vi "GenericProcess.vi"(11 "YTESTER测试数据":T1 caption="不要修改！") -> (3 "YTESTER结论":T2)   [LabVIEW 2017]
doc: "VIDescription=对某个变量进行判断的简单测试"
uses:
  YtCommon.lvlibp/yt`Step StepBaseInput.ctl
  YtCommon.lvlibp/yt`Step StepResult.ctl
  YtCommon.lvlibp/yt`Step TestData.ctl
  YtCommon.lvlibp/yt`Step System Queue.ctl
  Step`s VIs/YYLLGeneric/variable_W.ctl
  YtCommon.lvlibp/yt`Data-Ytester Type Data.ctl
  YtCommon.lvlibp
panel:
  in  "YTESTER开放参数":T4={"YTESTER_BaseInput"={"isTest"=FALSE, "isSkip"=FALSE, "StepName"="通用简易解析处理", "OnPass"=enum."Next", "OnFail"=enum."Next", "ReTestNumber"=0.0}, "数据源什么类型？"=enum."String类型", "String数据源"="", "NUM数据源"=0.0, "Bool数据源"=FALSE, "Smart预处理"=[], "解析后到变量(自定义建议#开头)"="#YtGenProcess1"}
  # "通用简易解析处理"
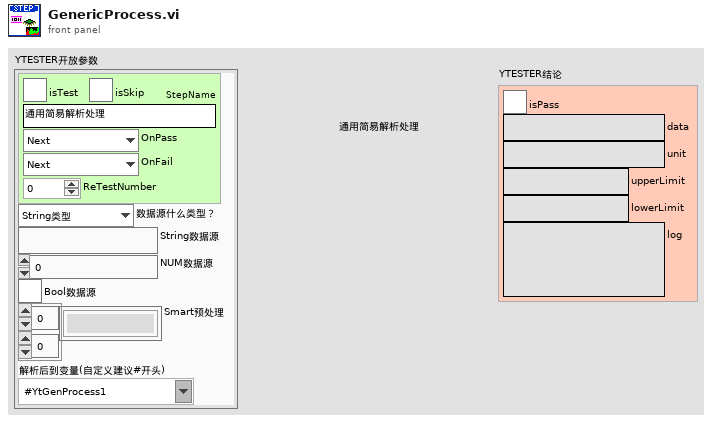
[diagram p1: front panel]
types:
  T1 = typedef "YtCommon.lvlibp/yt`Step TestData.ctl" = cluster{"Socket(From1)":i32, "SN":refnum<notifier>, "StopFlagRef":refnum<notifier>, "YT System Queue":refnum<queue>}
  T2 = typedef "YtCommon.lvlibp/yt`Step StepResult.ctl" = cluster{"isPass":bool, "data":string, "unit":string, "upperLimit":string, "lowerLimit":string, "log":string}
  T3 = typedef "YtCommon.lvlibp/yt`Step StepBaseInput.ctl" = cluster{"isTest":bool, "isSkip":bool, "StepName":string, "OnPass":enum16{"Next", "ToOVER", "Terminate"}, "OnFail":enum16{"Next", "ToOVER", "Terminate"}, "ReTestNumber":dbl}
  T4 = cluster{"YTESTER_BaseInput":T3, "数据源什么类型？":enum16{"String类型", "NUM类型", "Bool类型"}, "String数据源":string, "NUM数据源":dbl, "Bool数据源":bool, "Smart预处理":string[][], "解析后到变量(自定义建议#开头)":string}
  T5 = typedef "variable_W.ctl" = cluster{"YT_TYPE":T6, "TypeData":string[], "Tips":string}
  T6 = typedef "YtCommon.lvlibp/yt`Data-Ytester Type Data.ctl" = enum16{"NULL", "NUM", "BOOL", "TXT", "ENUM", "TIME", "PATH", "VISA", "COMBO", "ColorBox", "RadioBtn", "Array_NUM", "Array_BOOL", "Array_TXT", "Array_ENUM", "Array_PATH", "Array_COMBO"}
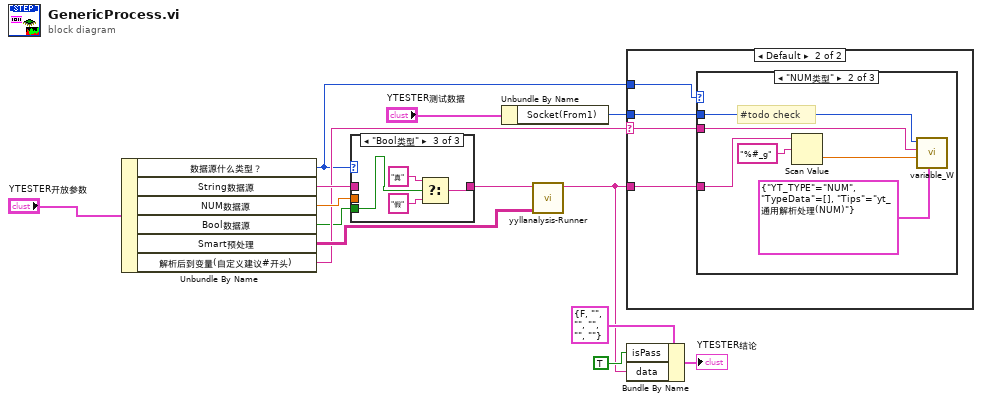
[diagram p0: block diagram]
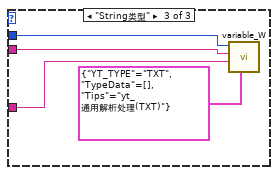
[diagram p4: hidden frame]
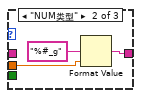
[diagram p6: hidden frame]
diagram:
  # "Y Y L L"
  n1 = Unbundle By Name("YTESTER开放参数") -> ("数据源什么类型？"=w3:enum16{"String类型", "NUM类型", "Bool类型"}, "String数据源"=w11:string, "NUM数据源"=w10:dbl, "Bool数据源"=w1:bool, "Smart预处理"=w8:string[][], "解析后到变量(自定义建议#开头)"=w6:string)
  n2 = case shown="\"Bool类型\"" w3 {
    tunnel: w11 -> [w15 _ _]
    tunnel: [w15 w17 w19] -> w9
    tunnel: w10 -> [_ w18 _]
    tunnel: w1 -> [_ _ w20]
    frame "String类型" {
    }
    frame "NUM类型" {
      n3 = Format Value(format string="%#_g", value (0)=w18) -> (output string=w17:string)  [unwired: 1 in]
    }
    frame "Bool类型" {
      n4 = Select(t="真", s=w20, f="假") -> (s? t:f=w19:string)
    }
  }
  n5 = Unbundle By Name("YTESTER测试数据") -> ("Socket(From1)"=w4:i32)
  n6 = call "yyllanalysis-Runner.vi"("inputs"=w8, "String in"=w9) -> ("String out"=w2:string)  [unwired: 8 in, 1 out]
  n7 = case shown="Default" w6 {
    selector: w6 -> [_ w25]
    tunnel: w4 -> [_ w26]
    tunnel: w3 -> [_ w24]
    tunnel: w2 -> [_ w23]
    frame "不到变量" {
    }
    frame Default {
      n8 = case shown="\"NUM类型\"" w24 {
        tunnel: w26 -> [_ w32 w36]
        tunnel: w25 -> [_ w31 w35]
        tunnel: w23 -> [_ w28 w33]
        frame Default {
        }
        frame "NUM类型" {
          # "#todo check"
          n9 = Scan Value(string=w28, format string="%#_g") -> (value=w29:dbl)  [unwired: 1 in, 1 out]
          n10 = call "variable_W.vi"("附加的Information"=T5 {"YT_TYPE"=enum."NUM", "TypeData"=[], "Tips"="yt_通用解析处理(NUM)"}, "待写入池的输入控件"=w29, "待写入池变量名称"=w31, "函数池名称 in"=w32) -> ()  [unwired: 5 in, 3 out]
        }
        frame "String类型" {
          n11 = call "variable_W.vi"("附加的Information"=T5 {"YT_TYPE"=enum."TXT", "TypeData"=[], "Tips"="yt_通用解析处理(TXT)"}, "待写入池的输入控件"=w33, "待写入池变量名称"=w35, "函数池名称 in"=w36) -> ()  [unwired: 5 in, 3 out]
        }
      }
    }
  }
  n12 = Bundle By Name(cluster=T2 {"isPass"=FALSE, "data"="", "unit"="", "upperLimit"="", "lowerLimit"="", "log"=""} ("Result"), "isPass"=TRUE, "data"=w2) -> (→"YTESTER结论":T2)
